vi "Set Output Range.vi"(8 "error in (no error)":errorcluster, 10 "output range":cluster{"output high":dbl, "output low":dbl}={"output high"=100.0, "output low"=-100.0} {"output low" format="%.2f"; "output high" format="%.2f"}, 11 "PID Loop in":refnum<class "PID Loop.lvclass">) -> (0 "error out":errorcluster, 3 "PID Loop out":refnum<class "PID Loop.lvclass">)   [LabVIEW 2024, in "PID Loop.lvlib" / "PID Loop.lvclass"]
uses:
  PID Loop.lvclass
  PID Loop.lvclass/PID Loop.ctl
  PID/PID/PID.lvclass
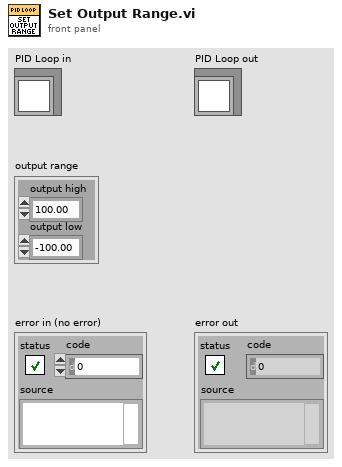
[diagram p1: front panel]
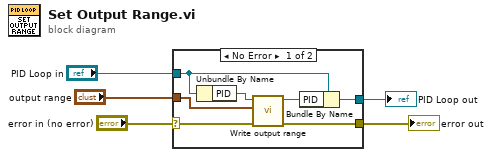
[diagram p0: block diagram]
diagram:
  n1 = case shown="No Error" "error in (no error)" {
    selector: "error in (no error)" -> [w10 w14]
    tunnel: [w9 w14] -> w4
    tunnel: [w7 w13] -> w2
    tunnel: "PID Loop in" -> [w8 w13]
    tunnel: "output range" -> [w11 _]
    frame No Error {
      n2 = Unbundle By Name(w8) -> ("PID"=w12:refnum<class "PID.lvclass">)
      n3 = call-dynamic "Write output range.vi"("error in (no error)"=w10, "output range"=w11, "PID in"=w12) -> ("error out"=w9:errorcluster, "PID out"=w6:refnum<class "PID.lvclass">)  [unwired: 7 in]
      n4 = Bundle By Name(cluster=w8, "PID"=w6) -> (w7:refnum<class "PID Loop.lvclass">)
    }
    frame Error {
    }
  }
  "error out" <- w4
  "PID Loop out" <- w2
